vi "inputFilter_aio.vi"(6 "Element in":cluster{"index":u16, "data":i16}, 7 "Output Valid":bool, 9 "aio.flt.p.b4x":fxp<+/-,24,8>[](array[numeric])=[0.0, 0.0, 0.0, 0.0, 0.0, 0.0, 0.0, 0.0, 0.0, 0.0, 0.0, 0.0], 10 "aio.flt.p.anot4x":fxp<+/-,24,8>[](array[numeric])=[0.0, 0.0, 0.0, 0.0, 0.0, 0.0, 0.0, 0.0], 11 "aio.flt.bypass":bool[](array[boolean])=[FALSE, FALSE, FALSE, FALSE]) -> (2 "output valid":bool, 3 "Element out":cluster{"index":u16, "y":fxp<+/-,20,17>} {"output" format="%.9g"})   [LabVIEW 2016]
uses:
  <vilib>/rvi/FXPMathLib/FxpInterpret/XNode/nifxpmath_Interpret.xnode
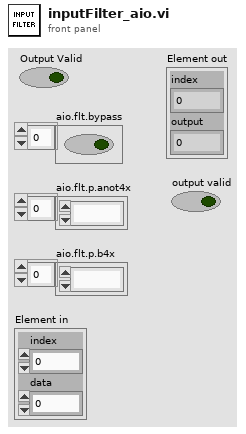
[diagram p1: front panel]
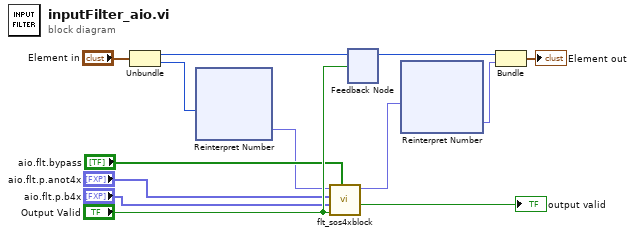
[diagram p0: block diagram]
diagram:
  n1 = Unbundle("Element in") -> ("index"=w11:u16, "data"=w4:i16)
  n2 = xnode "Reinterpret Number"("x"=w4) -> ("y"=w3:fxp<+/-,16,1>)
  n3 = call "flt_sos4xblock.vi"("sosBypass"="aio.flt.bypass", "input valid"="Output Valid", "b"="aio.flt.p.b4x", "anot"="aio.flt.p.anot4x", "input"=w3) -> ("output valid"=→"output valid":bool, "output"=w1:fxp<+/-,20,2>)  [unwired: 4 in, 1 out]
  n4 = feedback #1() -> (w12:u16)  [unwired: 1 in]
  n5 = feedback-in #1(w11, "Output Valid") -> ()
  n6 = xnode "Reinterpret Number"("x"=w1) -> ("y"=w2:fxp<+/-,20,17>)
  n7 = Bundle("index"=w12, "y"=w2) -> (→"Element out":cluster{"index":u16, "y":fxp<+/-,20,17>})  [unwired: 1 in]
